vi "FPGA Write FIFO - I32.vi"(6 "Timeout (ms)":u32, 8 "error in (no error)":errorcluster, 9 "Data":i32[](array[numeric]), 10 "FIFO":T1, 11 "FPGA Session In":refnum<class "Firmware Independent PID Interface.lvclass">) -> (0 "error out":errorcluster, 1 "Empty Elements Remaining":u32, 3 "FPGA Session Out":refnum<class "Firmware Independent PID Interface.lvclass">)   [LabVIEW 2010, in "Firmware Independent PID Interface.lvclass"]
doc: "Writes to a FIFO of signed 32-bit integers."
uses:
  Firmware Independent PID Interface.lvclass
  TypeDefs/HostToTargetFifoI32.ctl
  <vilib>/rvi/DataTransferAndStorage/Container/Common/niFpgaDataTypeControl.ctl
  <userlib>/_FPGA Interface Advanced Tools/FPGA Interface Base/FPGA Interface Base.lvclass/FPGA Interface Base.ctl
  <vilib>/Utility/error.llb/Error Cluster From Error Code.vi
  <userlib>/_FPGA Interface Advanced Tools/FPGA Interface Base/Accessors/FPGA Read Session.vi
  <userlib>/_FPGA Interface Advanced Tools/FPGA Interface Wrapper/FPGA Interface Wrapper.lvlib
  <userlib>/_FPGA Interface Advanced Tools/FPGA Interface Base/FPGA Interface Base.lvclass
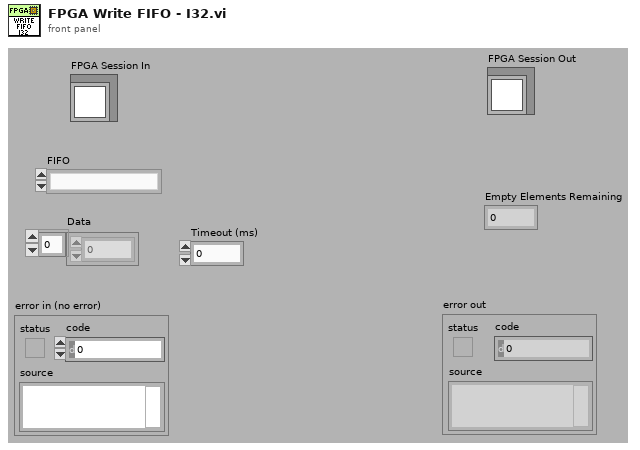
[diagram p1: front panel]
types:
  T1 = typedef "Firmware Independent PID Interface.lvclass/HostToTargetFifoI32.ctl" = enum16{""}
  T2 = typedef "niFpgaDataTypeControl.ctl" = enum32{"Boolean", "I8", "I16", "I32", "I64", "U8", "U16", "U32", "U64", "FXP", "CustomControl"}
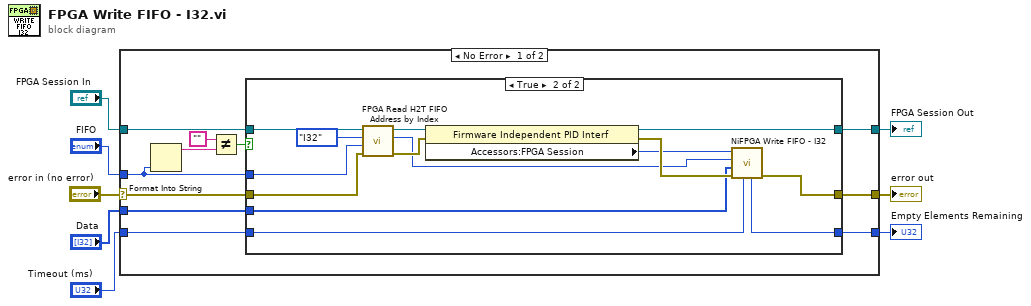
[diagram p0: block diagram]
diagram:
  n1 = case shown="No Error" "error in (no error)" {
    selector: "error in (no error)" -> [w9 w37]
    tunnel: [w11 w37] -> w2
    tunnel: [w12 w36] -> w3
    tunnel: "FPGA Session In" -> [w17 w36]
    tunnel: "FIFO" -> [w15 _]
    tunnel: [w10 _] -> w1
    tunnel: "Data" -> [w14 _]
    tunnel: "Timeout (ms)" -> [w13 _]
    frame No Error {
      n2 = Format Into String(w15) -> (resulting string=w19:string)  [unwired: 3 in, 1 out]
      n3 = Not Equal?(x="", y=w19) -> (x != y?=w16:bool)
      n4 = case shown="True" w16 {
        tunnel: [w20 w32] -> w11
        tunnel: [w21 w33] -> w12
        tunnel: w17 -> [w21 w31]
        tunnel: w15 -> [_ w29]
        tunnel: [_ w25] -> w10
        tunnel: w14 -> [_ w24]
        tunnel: w13 -> [_ w23]
        tunnel: w9 -> [w20 w22]
        frame False {
        }
        frame True {
          n5 = call <userlib>:"FPGA Read H2T FIFO Address by Index.vi"("error in (no error)"=w22, "index"=w29, "Data Type"=niFpgaDataTypeControl."I32", "FPGA Interface Base in"=w31) -> ("error out"=w27:errorcluster, "Address"=w26:u32, "FPGA Interface Base out"=w30:refnum<class "Firmware Independent PID Interface.lvclass">)  [unwired: 4 in, 1 out]
          n6 = property class="Firmware Independent PID Interf"(reference=w30, error in=w27) -> (reference out=w33:refnum<class "Firmware Independent PID Interface.lvclass">, error out=w35:errorcluster, "Accessors:FPGA Session"=w34:u32)
          n7 = call <userlib>:"NiFPGA Write FIFO - I32.vi"("Timeout"=w23, "error in (no error)"=w35, "Data"=w24, "FIFO"=w26, "Session"=w34) -> ("error out"=w32:errorcluster, "Empty Elements Remaining"=w25:u32)  [unwired: 4 in, 1 out]
        }
      }
    }
    frame Error {
    }
  }
  "error out" <- w2
  "FPGA Session Out" <- w3
  "Empty Elements Remaining" <- w1
